vi "Cap_File_Read.vi"(11 "Path":path) -> (2 "Capacitance (F)":dbl[](array[numeric]), 3 "Frequency (Hz)":dbl[](array[numeric]) format="%.2f")   [LabVIEW 2012]
uses:
  <vilib>/Utility/file.llb/Read From Spreadsheet File (string).vi
panel:
  out "C-F Graph":cluster{dbl[], dbl[]}(graph)
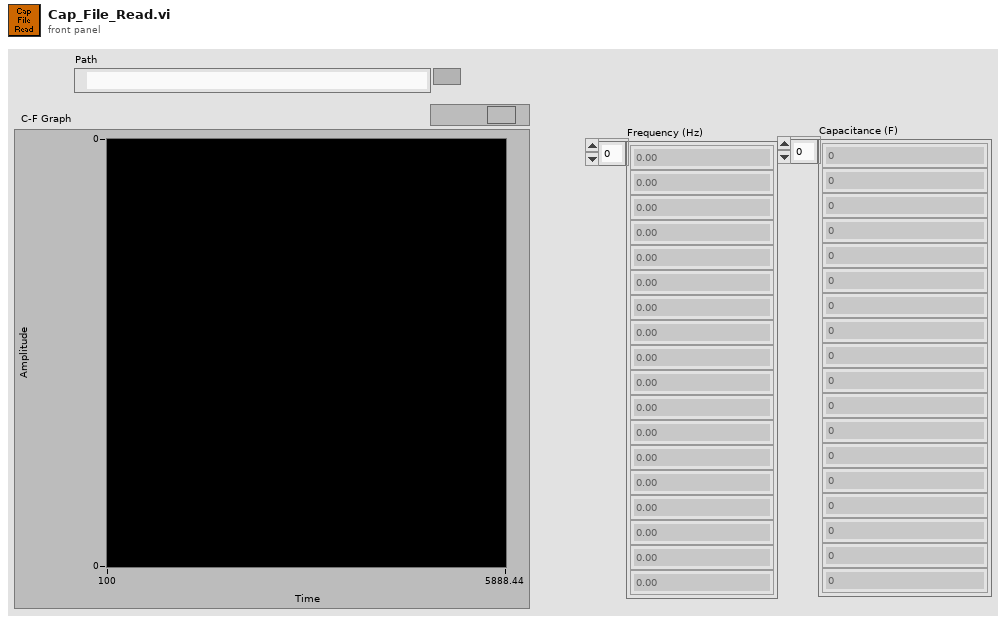
[diagram p1: front panel]
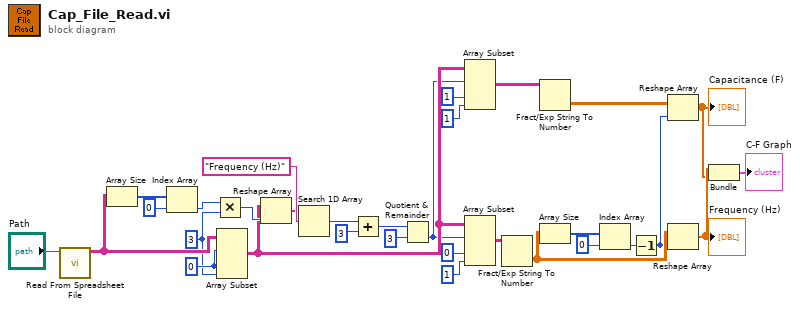
[diagram p0: block diagram]
diagram:
  w24 = 3
  w30 = 0 ("index")
  n1 = call-poly <vilib>:"Read From Spreadsheet File.vi"("file path (dialog if empty)"="Path") -> ("all rows"=w26:string[][])  [unwired: 6 in, 4 out]
  n2 = Array Size(array=w26) -> (size(s)=w27:i32[])
  n3 = Index Array(array=w27, index=0) -> (element=w29:i32)
  n4 = Multiply(x=w29, y=w24) -> (x*y=w25:i32)
  n5 = Array Subset(array=w26, index (row)=w30, index (col)=w30, length (col)=w24) -> (w10:string[][])  [unwired: 1 in]
  n6 = Reshape Array(w10, w25) -> (w11:string[])
  n7 = Search 1D Array(1D array=w11, element="Frequency (Hz)") -> (index of element=w19:i32)  [unwired: 1 in]
  n8 = Add(x=w19, y=3) -> (x+y=w21:i32)
  n9 = Quotient & Remainder(x=w21, y=3) -> (floor(x/y)=w9:i32)  [unwired: 1 out]
  n10 = Array Subset(array=w10, index (row)=w9, index (col)=1, length (col)=1) -> (w14:string[][])  [unwired: 1 in]
  n11 = Array Subset(array=w10, index (row)=w9, index (col)=0, length (col)=1) -> (w18:string[][])  [unwired: 1 in]
  n12 = Fract/Exp String To Number(string=w18) -> (number=w5:dbl[][])  [unwired: 3 in, 1 out]
  n13 = Fract/Exp String To Number(string=w14) -> (number=w15:dbl[][])  [unwired: 3 in, 1 out]
  n14 = Array Size(array=w5) -> (size(s)=w8:i32[])
  n15 = Index Array(array=w8, index=0) -> (element=w6:i32)
  n16 = Decrement(x=w6) -> (x-1=w4:i32)
  n17 = Reshape Array(w15, w4) -> (w2:dbl[])
  "Capacitance (F)" <- w2
  n18 = Reshape Array(w5, w4) -> (w3:dbl[])
  "Frequency (Hz)" <- w3
  n19 = Bundle(w3, w2) -> (→"C-F Graph":cluster{dbl[], dbl[]})  [unwired: 1 in]
